vi "Confirm Shutdown.vi"(8 "error in (no error)":errorcluster, 11 "controller queue":refnum<queue>) -> (0 "error out":errorcluster)   [LabVIEW 2020]
uses:
  Controller Loop/Message and Data.ctl
  Inflation Test/Parameter Class/IA Test Parameters.lvclass
  Controllers/Controller.lvclass
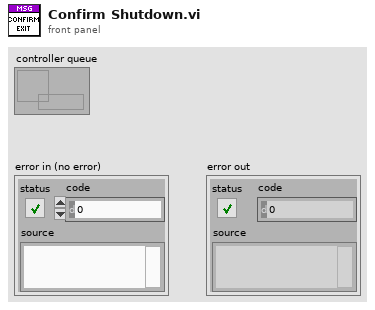
[diagram p1: front panel]
types:
  T1 = typedef "Message and Data.ctl" = cluster{"msg":string, "ia test param":refnum<class "IA Test Parameters.lvclass">, "controller type":refnum<class "Controller.lvclass">, "folder path":path, "file name":string}
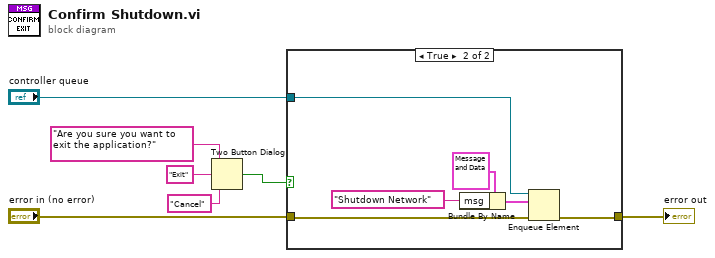
[diagram p0: block diagram]
diagram:
  n1 = Two Button Dialog(message="Are you sure you want to exit the application?", 1:"Cancel" ("F button name (\"Cancel\")"), 2:"Exit" ("T button name (\"OK\")")) -> (T button?=w7:bool)
  n2 = case shown="True" w7 {
    tunnel: "controller queue" -> [_ w14]
    tunnel: "error in (no error)" -> [w8 w10]
    tunnel: [w8 w9] -> w6
    frame False {
    }
    frame True {
      n3 = Bundle By Name(cluster=T1 {"msg"="", "ia test param"=refnum, "controller type"=refnum, "folder path"=path "", "file name"=""} ("element"), "msg"="Shutdown Network") -> (w12:T1)
      n4 = Enqueue Element(queue=w14, element=w12, error in (no error)=w10) -> (error out=w9:errorcluster)  [unwired: 1 in, 2 out]
    }
  }
  "error out" <- w6
